vi "Configure.vi"(8 "error in":errorcluster, 10 "name":string="ePAS", 11 "ePAS in":refnum<class "ePAS.lvclass">) -> (0 "error out":errorcluster, 3 "ePAS out":refnum<class "ePAS.lvclass">)   [LabVIEW 2014, in "ePAS Library.lvlib" / "ePAS.lvclass"]
doc: "Configure the instrument class. If there is no config file specified, an error"
uses:
  ePAS.lvclass
  FPGA/Session/Exscalabar FPGA.lvclass
  Commands/Change Laser Voffset/Change Laser Voffset.lvclass
  Commands/Change Laser Modulation/Change Laser Modulation.lvclass
  Commands/Change Laser Vrange/Change Laser Vrange.lvclass
  Commands/Change PAS Laser Frequency/Change Laser Frequency.lvclass
  Commands/Copy of Change Laser Enable State/Change Laser Enable State.lvclass
  Commands/Change Speaker State/Change Speaker State.lvclass
  Commands/Change Speaker Switch State/Change Speaker Switch State.lvclass
  Commands/Change Speaker Vparams/Change Speaker Vparams.lvclass
  Commands/Change iSpk Signal/Change iSpk Signal.lvclass
  reusable/Instrument/Instrument.lvclass/Instrument.ctl
  FPGA/Session/Exscalabar FPGA.lvclass/Exscalabar FPGA.ctl
  reusable/Session APIs/File Access/Config Data/Config Data.lvclass/Config Data.ctl
  Commands/Change Laser Voffset/Change Laser Voffset.lvclass/Change Laser Voffset.ctl
  Commands/Change Laser Vrange/Change Laser Vrange.lvclass/Change Laser Vrange.ctl
  Commands/Change PAS Laser Frequency/Change Laser Frequency.lvclass/Change Laser Frequency.ctl
  Commands/Copy of Change Laser Enable State/Change Laser Enable State.lvclass/Change Laser Enable State.ctl
  Commands/Change iSpk Signal/Change iSpk Signal.lvclass/Change iSpk Signal.ctl
  Commands/Change Speaker Switch State/Change Speaker Switch State.lvclass/Change Speaker Switch State.ctl
  Commands/Change Speaker Vparams/Change Speaker Vparams.lvclass/Change Speaker Vparams.ctl
  Commands/Change Laser Modulation/Change Laser Modulation.lvclass/Change Laser Modulation.ctl
  ePAS.lvclass/ePAS.ctl
  reusable/Session APIs/File Access/Config Data/Accessors/Read Ref.vi
  reusable/Instrument/Read Log Session.vi
  reusable/Instrument/Read Cfg Session.vi
  reusable/Instrument/Read CMD.vi
  Commands/Change Speaker Switch State/Write Length.vi
  Commands/Change Speaker Switch State/Write Period.vi
  Commands/Change Speaker Switch State/Write Cycle.vi
  FPGA/Session/Write logSession.vi
  FPGA/Session/Write configSession.vi
  reusable/Session APIs/File Access/Config Data/Read Array/Read Boolean Array.vi
  reusable/Session APIs/File Access/Config Data/Read Array/Read DBL Array.vi
  reusable/Session APIs/File Access/Config Data/Read Array/Read String Array.vi
  <vilib>/Utility/config.llb/Read Key (Boolean).vi
  <vilib>/Utility/config.llb/Read Key (I32).vi
  <vilib>/Utility/config.llb/Read Key (Double).vi
  reusable/PAS/Main/PAS.lvclass
  <userlib>/_Session Fwk/Session - Root.lvclass
  reusable/Session APIs/File Access/Config Data/Config Data.lvclass
  reusable/Command/Command.lvclass
  reusable/Session APIs/Session Log/System Log.lvclass
  <vilib>/Utility/config.llb/NI_LVConfig.lvlib
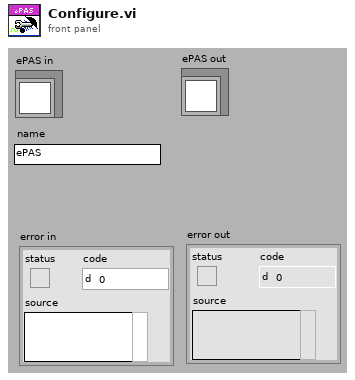
[diagram p1: front panel]
types:
  T1 = typedef "Session - Root.lvclass/Session Handle.ctl" = refnum<data-value>
  T2 = typedef "Config Data.lvclass/Config Session.ctl" = refnum<data-value>
  T3 = typedef "NI_LVConfig.lvlib/Config Data RefNum.ctl" = refnum<k1>
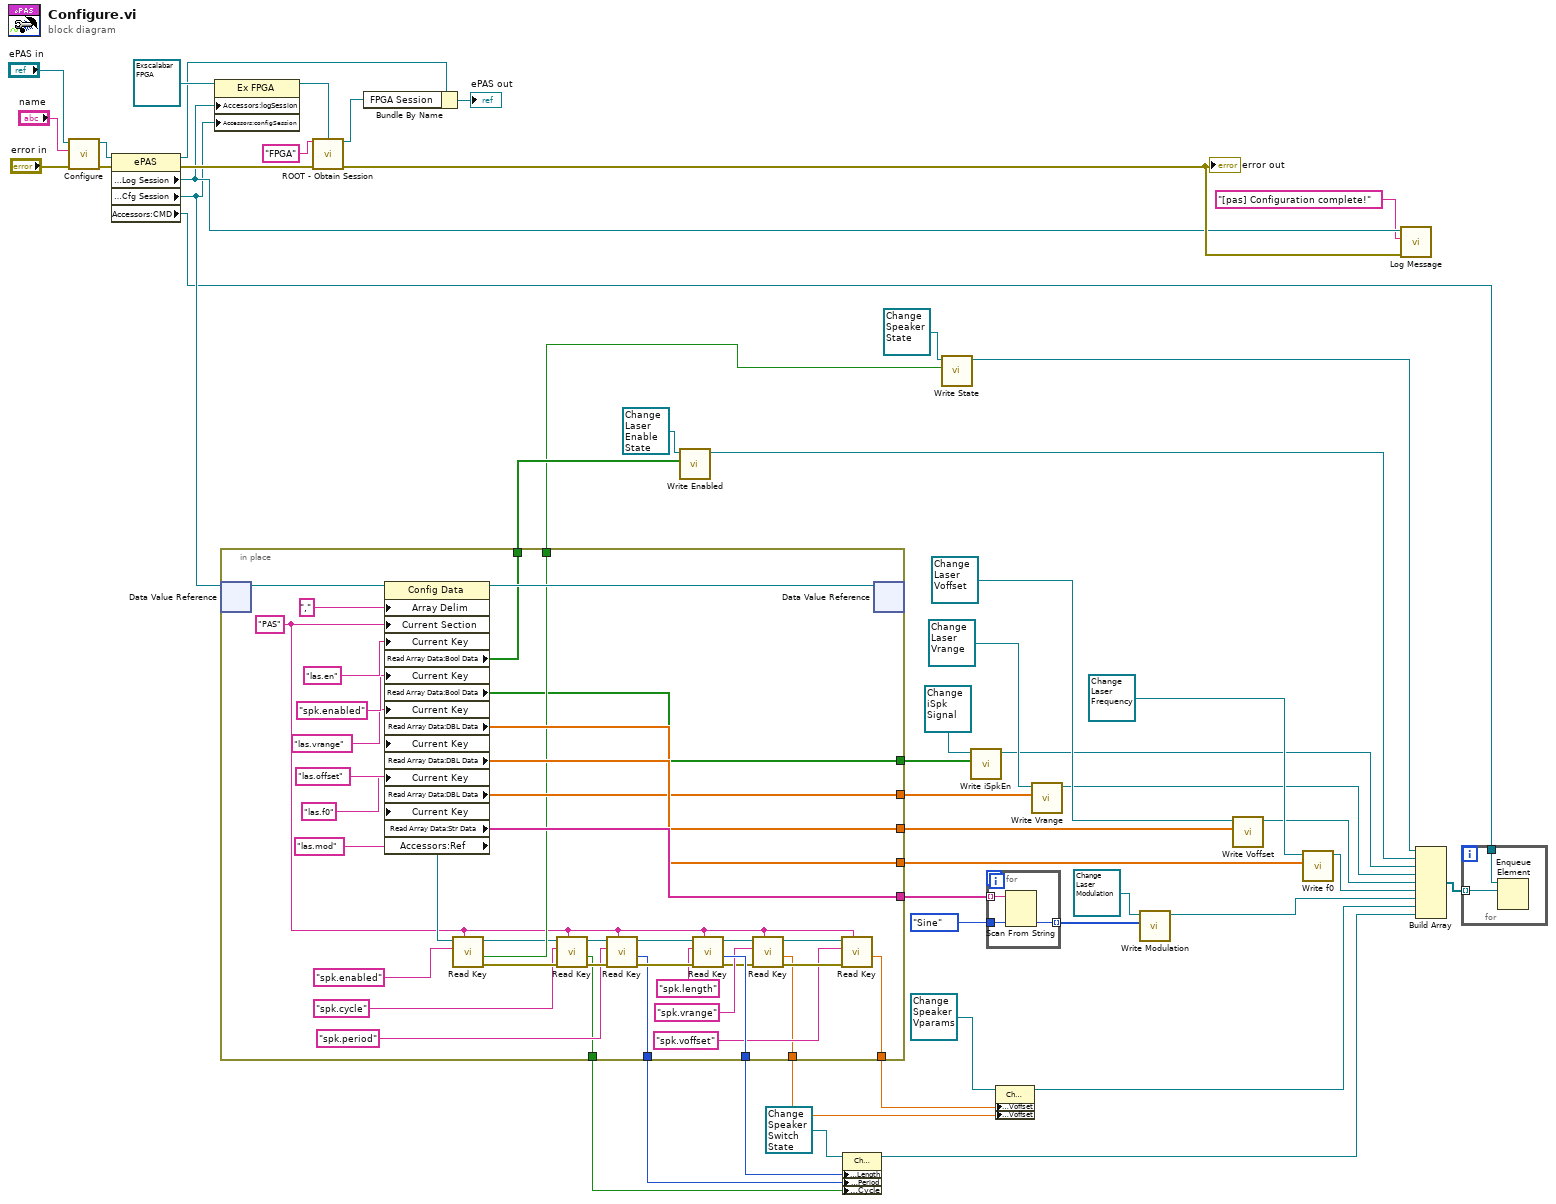
[diagram p0: block diagram]
diagram:
  n1 = call-parent "Configure.vi"("error in"="error in", "name"="name", "PAS in"="ePAS in") -> ("error out"=w38:errorcluster, "PAS out"=w46:refnum<class "ePAS.lvclass">)  [unwired: 7 in]
  n2 = property class="ePAS"(reference=w46, error in=w38) -> (reference out=w42:refnum<class "ePAS.lvclass">, error out=w39:errorcluster, "Accessors:Log Session"=w37:T1, "Accessors:Cfg Session"=w35:T2, "Accessors:CMD"=w24:refnum<queue>)
  n3 = property class="Ex FPGA"(reference=refnum<class "Exscalabar FPGA.lvclass"> refnum ("Ex FPGA"), "Accessors:logSession"=w37, "Accessors:configSession"=w35) -> (reference out=w44:refnum<class "Exscalabar FPGA.lvclass">)  [unwired: 1 in, 1 out]
  n4 = in-place {
    in-place-border: [w80] -> w34
    in-place-border: [w79] -> w13
    in-place-border: [w78] -> w30
    in-place-border: [w77] -> w27
    in-place-border: [w76] -> w25
    in-place-border: [w73] -> w21
    in-place-border: [w63] -> w19
    in-place-border: [w62] -> w12
    in-place-border: [w61] -> w18
    in-place-border: [w54] -> w10
    in-place-border: [w53] -> w11
    in-place-border: [w52] -> w14
    w56 = "PAS" ("Current Section")
    n5 = in-place-dvr #1(w35) -> (w89:refnum<class "Config Data.lvclass">)  [unwired: 1 out]
    n6 = property class="Config Data"(reference=w89, "Array Delim"=",", "Current Section"=w56, "Current Key"="las.en", "Current Key"="spk.enabled", "Current Key"="las.vrange", "Current Key"="las.offset", "Current Key"="las.f0", "Current Key"="las.mod") -> (reference out=w85:refnum<class "Config Data.lvclass">, "Read Array Data:Bool Data"=w76:bool[], "Read Array Data:Bool Data"=w52:bool[], "Read Array Data:DBL Data"=w78:dbl[], "Read Array Data:DBL Data"=w79:dbl[], "Read Array Data:DBL Data"=w77:dbl[], "Read Array Data:Str Data"=w80:string[], "Accessors:Ref"=w75:T3)  [unwired: 1 in, 1 out]
    n7 = call-poly <vilib>:"Read Key.vi"("section"=w56, "key"="spk.enabled", "refnum"=w75) -> ("error out"=w71:errorcluster, "value"=w73:bool, "refnum out"=w72:T3)  [unwired: 5 in, 1 out]
    n8 = call-poly <vilib>:"Read Key.vi"("section"=w56, "error in (no error)"=w71, "key"="spk.cycle", "refnum"=w72) -> ("error out"=w69:errorcluster, "value"=w62:bool, "refnum out"=w70:T3)  [unwired: 4 in, 1 out]
    n9 = call-poly <vilib>:"Read Key.vi"("section"=w56, "error in (no error)"=w69, "key"="spk.period", "refnum"=w70) -> ("error out"=w67:errorcluster, "value"=w61:i32, "refnum out"=w68:T3)  [unwired: 4 in, 1 out]
    n10 = call-poly <vilib>:"Read Key.vi"("section"=w56, "error in (no error)"=w67, "key"="spk.length", "refnum"=w68) -> ("error out"=w51:errorcluster, "value"=w63:i32, "refnum out"=w60:T3)  [unwired: 4 in, 1 out]
    n11 = call-poly <vilib>:"Read Key.vi"("section"=w56, "error in (no error)"=w51, "key"="spk.vrange", "refnum"=w60) -> ("error out"=w57:errorcluster, "value"=w54:dbl, "refnum out"=w58:T3)  [unwired: 4 in, 1 out]
    n12 = call-poly <vilib>:"Read Key.vi"("section"=w56, "error in (no error)"=w57, "key"="spk.voffset", "refnum"=w58) -> ("value"=w53:dbl)  [unwired: 4 in, 3 out]
    n13 = in-place-dvr #1(w85) -> ()  [unwired: 2 out]
  }
  n14 = call <userlib>:"ROOT - Obtain Session.vi"("Session Name ()"="FPGA", "OBJ - Session"=w44, "error in (no error)"=w39) -> ("Session Handle"=w41:T1, "error out"=w43:errorcluster)  [unwired: 10 in, 1 out]
  "error out" <- w43
  n15 = Bundle By Name(cluster=w42, "FPGA Session"=w41) -> (→"ePAS out":refnum<class "ePAS.lvclass">)
  n16 = call "Write Enabled.vi"("Enabled?"=w25, "Change Laser Frequency in"=refnum<class "Change Laser Enable State.lvclass"> refnum ("Change Laser Enable State.lvclass")) -> ("Change Laser Frequency out"=w2:refnum<class "Change Laser Enable State.lvclass">)  [unwired: 8 in, 1 out]
  n17 = property class="Change Speaker Switch"(reference=refnum<class "Change Speaker Switch State.lvclass"> refnum ("Change Speaker Switch"), "Accessors:Length"=w19, "Accessors:Period"=w18, "Accessors:Cycle"=w12) -> (reference out=w8:refnum<class "Change Speaker Switch State.lvclass">)  [unwired: 1 in, 1 out]
  n18 = call "Write State.vi"("State"=w21, "Change Speaker State in"=refnum<class "Change Speaker State.lvclass"> refnum ("Change Speaker State")) -> ("Change Speaker State out"=w1:refnum<class "Change Speaker State.lvclass">)  [unwired: 8 in, 1 out]
  n19 = call "Write iSpkEn.vi"("iSpkEn"=w14, "Change iSpkEn in"=refnum<class "Change iSpk Signal.lvclass"> refnum ("Change iSpk Signal.lvclass")) -> ("Change iSpkEn out"=w3:refnum<class "Change iSpk Signal.lvclass">)  [unwired: 8 in, 1 out]
  n20 = for {
    tunnel: w34 -> [w92] mode=indexing
    tunnel: [w91] -> w32 mode=indexing
    tunnel: enum8{"Sine", "Square"}."Sine" ("Mod") -> [w90]
    n21 = Scan From String(input string=w92, default 1=w90) -> (output 1=w91:enum8{"Sine", "Square"})  [unwired: 3 in, 3 out]
  }
  n22 = property class="Change Speaker Vparams"(reference=refnum<class "Change Speaker Vparams.lvclass"> refnum ("Change Speaker Vparams"), "Accessors:Voffset"=w11, "Accessors:Voffset"=w10) -> (reference out=w16:refnum<class "Change Speaker Vparams.lvclass">)  [unwired: 1 in, 1 out]
  n23 = call "Write Vrange.vi"("Vrange"=w30, "Change Laser Frequency in"=refnum<class "Change Laser Vrange.lvclass"> refnum) -> ("Change Laser Frequency out"=w4:refnum<class "Change Laser Vrange.lvclass">)  [unwired: 8 in, 1 out]
  n24 = call "Write Modulation.vi"("Modulation"=w32, "Change Laser Frequency in"=refnum<class "Change Laser Modulation.lvclass"> refnum) -> ("Change Laser Frequency out"=w7:refnum<class "Change Laser Modulation.lvclass">)  [unwired: 8 in, 1 out]
  n25 = call "Write Voffset.vi"("Voffset"=w13, "Change Laser Frequency in"=refnum<class "Change Laser Voffset.lvclass"> refnum ("Change Laser Voffset.lvclass")) -> ("Change Laser Frequency out"=w5:refnum<class "Change Laser Voffset.lvclass">)  [unwired: 8 in, 1 out]
  n26 = call "Write f0.vi"("f0"=w27, "Change Laser Frequency in"=refnum<class "Change Laser Frequency.lvclass"> refnum ("Change Laser Frequency.lvclass")) -> ("Change Laser Frequency out"=w6:refnum<class "Change Laser Frequency.lvclass">)  [unwired: 8 in, 1 out]
  n27 = call "Log Message.vi"("error in"=w43, "MSG In"="[pas] Configuration complete!", "session in"=w37) -> ()  [unwired: 7 in, 2 out]
  n28 = Build Array(w1, w2, w3, w4, w5, w6, w7, w16, w8) -> (w23:refnum<class "Command.lvclass">[])
  n29 = for {
    tunnel: w24 -> [w94]
    tunnel: w23 -> [w93] mode=indexing
    n30 = Enqueue Element(queue=w94, element=w93) -> ()  [unwired: 2 in, 3 out]
  }
